vi "SendDBL.vi"(8 "error in (no error)":errorcluster, 10 "In":dbl, 11 "reference in":refnum<class "PerformanceTest.lvclass">) -> (0 "error out":errorcluster, 2 "Out":dbl, 3 "reference out":refnum<class "PerformanceTest.lvclass">)   [LabVIEW 2018, in "PerformanceTest.lvclass"]
uses:
  PerformanceTest.lvclass
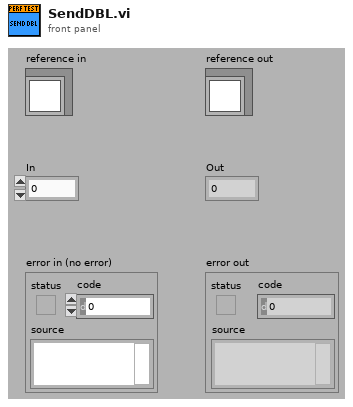
[diagram p1: front panel]
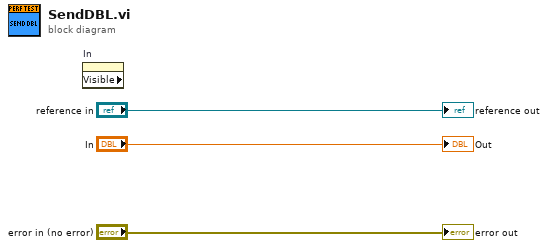
[diagram p0: block diagram]
diagram:
  n1 = property on="In" class="DigNum (strict)" props=["Visible"]() -> ()  [unwired: 2 in, 3 out]
  "error out" <- "error in (no error)"
  "reference out" <- "reference in"
  "Out" <- "In"
